vi "controller FG.vi"(9 "Enum":enum16{"get", "set", "release"}(ring), 10 "Sensor Sim Timing":T1=[{"Station"=enum."Entry", "Wash Step"=enum."None", "Step Time"=0.0}, {"Station"=enum."Station 1", "Wash Step"=enum."Under Body Wash", "Step Time"=30.0}, {"Station"=enum."Station 1", "Wash Step"=enum."Bug Remover", "Step Time"=20.0}, {"Station"=enum."Station 2", "Wash Step"=enum."Pre-Soak", "Step Time"=50.0}, {"Station"=enum."Station 2", "Wash Step"=enum."High Pressure Wash", "Step Time"=60.0}, {"Station"=enum."Station 2", "Wash Step"=enum."Low Pressure Wax", "Step Time"=45.0}, {"Station"=enum."Station 2", "Wash Step"=enum."Spot Free Rinse", "Step Time"=50.0}, {"Station"=enum."Station 3", "Wash Step"=enum."Tire Shine", "Step Time"=45.0}, {"Station"=enum."Station 3", "Wash Step"=enum."Air Dry", "Step Time"=50.0}, {"Station"=enum."Exit", "Wash Step"=enum."None", "Step Time"=0.0}]) -> ()   [LabVIEW 2018]
doc: "store vehcile position array from VPS module"
uses:
  Vehicle Position Simulator/Public Controls/Sensor Sim Array.ctl
  Vehicle Position Simulator/Public Controls/Sensor SIm Timing.ctl
panel:
  out "Sensor Sim Timing out":T1=[{"Station"=enum."Entry", "Wash Step"=enum."None", "Step Time"=0.0}, {"Station"=enum."Station 1", "Wash Step"=enum."Under Body Wash", "Step Time"=30.0}, {"Station"=enum."Station 1", "Wash Step"=enum."Bug Remover", "Step Time"=20.0}, {"Station"=enum."Station 2", "Wash Step"=enum."Pre-Soak", "Step Time"=50.0}, {"Station"=enum."Station 2", "Wash Step"=enum."High Pressure Wash", "Step Time"=60.0}, {"Station"=enum."Station 2", "Wash Step"=enum."Low Pressure Wax", "Step Time"=45.0}, {"Station"=enum."Station 2", "Wash Step"=enum."Spot Free Rinse", "Step Time"=50.0}, {"Station"=enum."Station 3", "Wash Step"=enum."Tire Shine", "Step Time"=45.0}, {"Station"=enum."Station 3", "Wash Step"=enum."Air Dry", "Step Time"=50.0}, {"Station"=enum."Exit", "Wash Step"=enum."None", "Step Time"=0.0}]
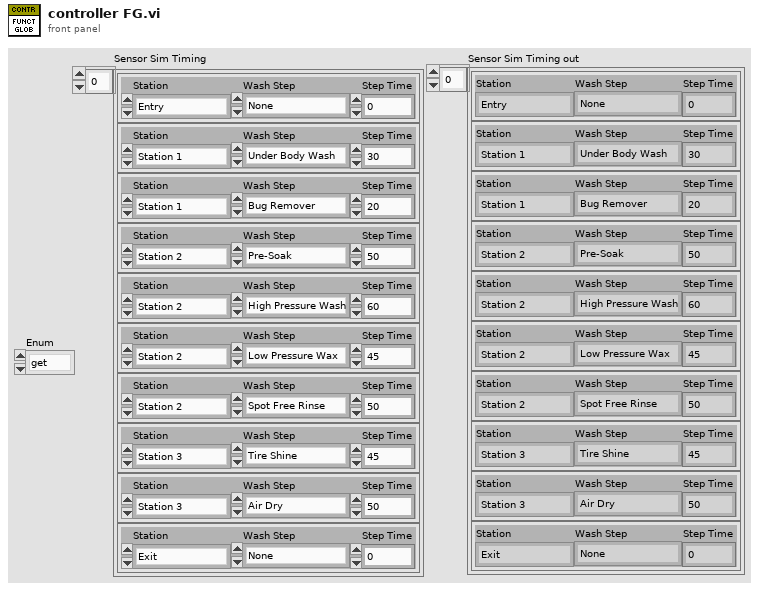
[diagram p1: front panel]
types:
  T1 = typedef "Vehicle Position Interface Simulator.lvlib/Sensor Sim Array.ctl" = T2[]
  T2 = typedef "Vehicle Position Interface Simulator.lvlib/Sensor SIm Timing.ctl" = cluster{"Station":enum16{"Entry", "Station 1", "Station 2", "Station 3", "Exit", "Out of Position"}, "Wash Step":enum16{"None", "Under Body Wash", "Bug Remover", "Pre-Soak", "High Pressure Wash", "Low Pressure Wax", "Spot Free Rinse", "Tire Shine", "Air Dry", ""}, "Step Time":dbl}
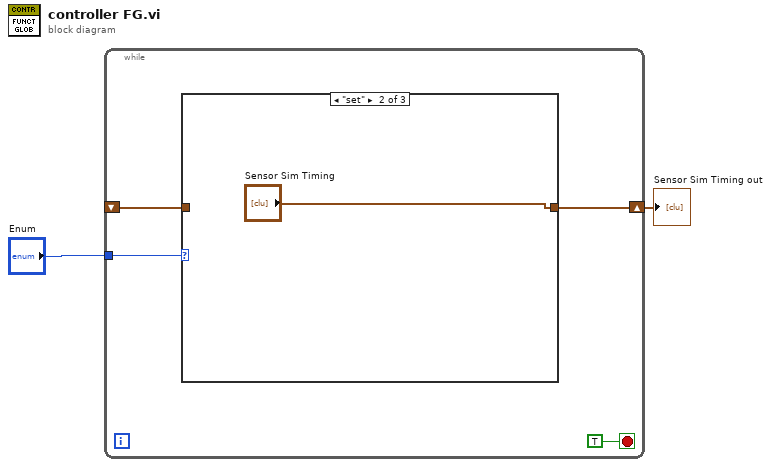
[diagram p0: block diagram]
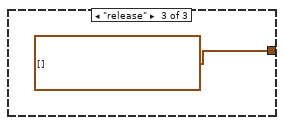
[diagram p3: hidden frame]
diagram:
  n1 = while {
    tunnel: "Enum" -> [w6]
    shift-right: [w4] -> w1
    shift-left: _ -> [w5]
    stop <- TRUE stop-if-true
    n2 = case shown="\"set\"" w6 {
      tunnel: w5 -> [w7 _ _]
      tunnel: [w7 "Sensor Sim Timing" T1 [] ("Sensor Sim Timing")] -> w4
      frame "get", Default {
      }
      frame "set" {
      }
      frame "release" {
      }
    }
  }
  "Sensor Sim Timing out" <- w1
